vi "MainProgressBar.vi"() -> ()   [LabVIEW 2019]
panel:
  out "滑动杆":dbl(slide) scale=0.0..10.0
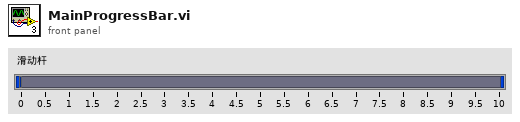
[diagram p1: front panel]
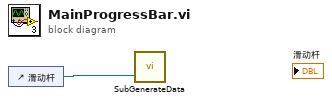
[diagram p0: block diagram]
diagram:
  n1 = control-ref of="滑动杆"() -> (w1:refnum<vi>)
  n2 = call "SubGenerateData.vi"("Slide引用句柄"=w1) -> ()  [unwired: 2 in, 1 out]
